vi "Acquire Data.vi"(8 "error in (no error)":errorcluster, 11 "Simulated Camera in":refnum<class "Simulated Camera.lvclass">) -> (0 "error out":errorcluster, 3 "Simulated Camera out":refnum<class "Simulated Camera.lvclass">)   [LabVIEW 2020, in "Simulated Camera.lvclass"]
uses:
  Simulated Camera.lvclass
  Simulated Camera.lvclass/Simulated Camera.ctl
  General Hardware.lvclass
  Camera.lvclass
  <vilib>/vision/Image Controls.llb/IMAQ Image.ctl
  C:/Users/jharw/Documents/1 Folder to Rule them All/UMD/Inflation-Apparatus/src/Hardware/General Hardware.lvclass
  C:/Users/jharw/Documents/1 Folder to Rule them All/UMD/Inflation-Apparatus/src/Hardware/Sensors/Cameras/Camera.lvclass
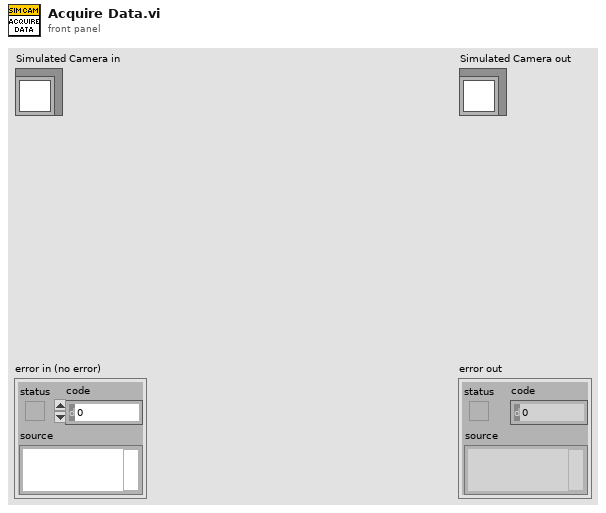
[diagram p1: front panel]
types:
  T1 = typedef "IMAQ Image.ctl" = refnum<image>
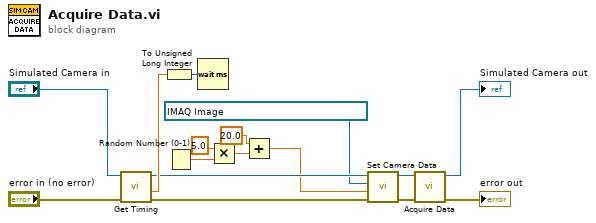
[diagram p0: block diagram]
diagram:
  n1 = call "Get Timing.vi"("error in (no error)"="error in (no error)", "General Hardware in"="Simulated Camera in") -> ("error out"=w12:errorcluster, "time delay (ms)"=w13:dbl, "General Hardware out"=w7:refnum<class "Simulated Camera.lvclass">)  [unwired: 6 in, 1 out]
  n2 = To Unsigned Long Integer(number=w13) -> (unsigned 32bit integer=w14:u32)
  n3 = Random Number (0-1)() -> (number: 0 to 1=w11:dbl)
  n4 = Wait (ms)(milliseconds to wait=w14) -> ()  [unwired: 1 out]
  n5 = Multiply(x=5.0, y=w11) -> (x*y=w9:dbl)
  n6 = Add(x=20.0, y=w9) -> (x+y=w6:dbl)
  n7 = call "Set Camera Data.vi"("error in (no error)"=w12, "diameter (mm)"=w6, "image"=T1 refnum ("current image"), "Camera in"=w7) -> ("error out"=w3:errorcluster, "Camera out"=w4:refnum<class "Simulated Camera.lvclass">)  [unwired: 6 in]
  n8 = call-parent "Acquire Data.vi"("error in (no error)"=w3, "Camera in"=w4) -> ("error out"=→"error out":errorcluster, "Camera out"=→"Simulated Camera out":refnum<class "Simulated Camera.lvclass">)  [unwired: 8 in]
